vi "Add_degrees_wraparound.vi"(1 "DEG 2":dbl, 2 "DEG 1":dbl) -> (0 "DEG OUT":dbl)   [LabVIEW 2019]
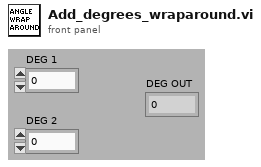
[diagram p1: front panel]
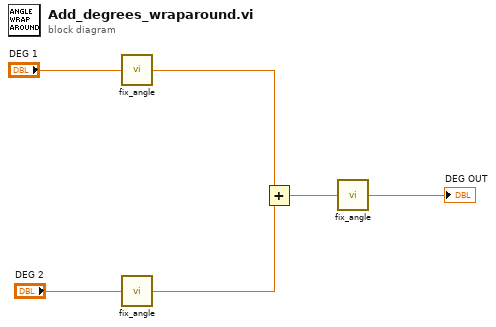
[diagram p0: block diagram]
diagram:
  n1 = call "fix_angle.vi"("Angle IN"="DEG 1") -> ("Angle OUT"=w4:dbl)  [unwired: 4 in]
  n2 = call "fix_angle.vi"("Angle IN"="DEG 2") -> ("Angle OUT"=w3:dbl)  [unwired: 4 in]
  n3 = Add(x=w4, y=w3) -> (x+y=w2:dbl)
  n4 = call "fix_angle.vi"("Angle IN"=w2) -> ("Angle OUT"=→"DEG OUT":dbl)  [unwired: 4 in]
